vi "Configure FPGA.vi"   [LabVIEW 2015, in "Fuel Injection Addon Engine.lvlib"]
uses:
  Fuel Injection Addon Engine.lvlib
  <vilib>/rvi/interface/nirviReadWriteControl/nirviReadWriteControl.xnode
  Types/FPGA Reference.ctl
  <vilib>/Utility/error.llb/Error Cluster From Error Code.vi
  <vilib>/rvi/interface/Simulation/niFpgaSimulationCallBeginRW.vi
  <vilib>/rvi/errors/niLvFpgaAdjustHostInterfaceError.vi
  <vilib>/NI Veristand/Custom Device Tools/Custom Device Utility Library/Custom Device Utility Library.lvlib
  NiFpgaLv.dll
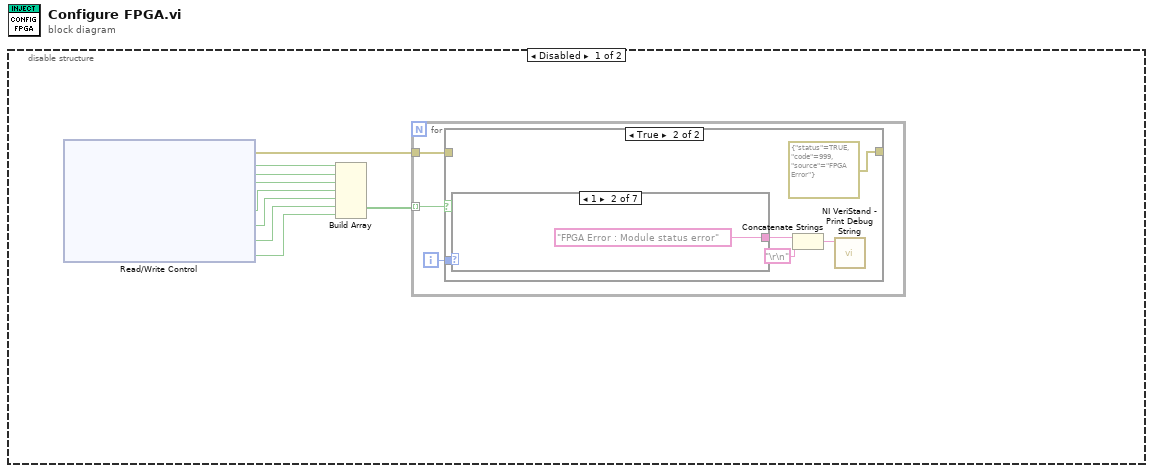
[diagram p0: block diagram]
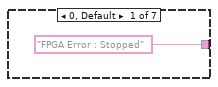
[diagram p3: hidden frame]
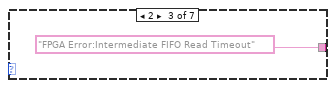
[diagram p4: hidden frame]
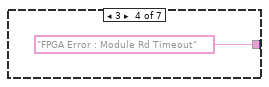
[diagram p5: hidden frame]
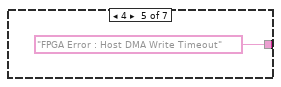
[diagram p6: hidden frame]
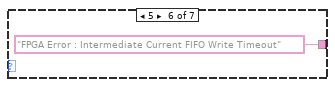
[diagram p7: hidden frame]
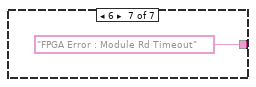
[diagram p8: hidden frame]
diagram:
  n1 = disable-structure shown="Disabled" {
    frame Disabled {
      n2 = xnode "Read/Write Control"() -> ("error out"=w7:errorcluster, "Stopped"=w9:bool, "Module status error"=w2:bool, "Intermediate FIFO Rd Timeout"=w6:bool, "Module Rd Timeout"=w5:bool, "Host DMA Timeout"=w4:bool, "Intermediate FIFO Write Timeout"=w3:bool, "Module Rd Timeout"=w1:bool)  [unwired: 2 in, 1 out]
      n3 = Build Array(w9, w2, w6, w5, w4, w3, w1) -> (w8:bool[])
      n4 = for {
        tunnel: w8 -> [w12] mode=indexing
        tunnel: w7 -> [w10]
        i -> [w11]
        n5 = case shown="True" w12 {
          tunnel: w11 -> [_ w18]
          tunnel: w10 -> [w13 _]
          tunnel: [w13 errorcluster {"status"=TRUE, "code"=999, "source"="FPGA Error"} ("error constant")] -> _
          frame False {
          }
          frame True {
            n6 = case shown="1" w18 {
              tunnel: ["FPGA Error : Stopped" ("string") "FPGA Error : Module status error" ("string") "FPGA Error:Intermediate FIFO Read Timeout" ("string") "FPGA Error : Module Rd Timeout" ("string") "FPGA Error : Host DMA Write Timeout" ("string") "FPGA Error : Intermediate Current FIFO Write Timeout" ("string") "FPGA Error : Module Rd Timeout" ("string")] -> w15
              frame 0, Default {
              }
              frame 1 {
              }
              frame 2 {
              }
              frame 3 {
              }
              frame 4 {
              }
              frame 5 {
              }
              frame 6 {
              }
            }
            n7 = Concatenate Strings(w15, "\r\n") -> (w17:string)
            n8 = call <vilib>:"NI VeriStand - Print Debug String.vi"("Message"=w17) -> ()  [unwired: 10 in, 1 out]
          }
        }
      }
    }
    frame Enabled {
    }
  }
